vi "Main.vi"(10 "DAQ Type":enum16{"Hardware", "Simulation"}(ring), 11 "Module Admin":refnum<class "Delacor_lib_QMH_Module Admin.lvclass">) -> ()   [LabVIEW 2016, in "Environment Chamber.lvlib"]
doc: "This template is based off of the Queued Message Handler design pattern and the Queued Message Handler project template that ships with LabVIEW.\n\nThe main difference is that the queue is private to this module and communication between modules is performed via Broadcast and Request events.\n\nRequest events are wrapped in public API methods and are handled in the Event Handling Loop (EHL) of this VI. Any module can register for Broadcast events sent by this module. The EHL generates messages based on user interface actions.\n\nThe Message Handling Loop (MHL) processes messages generated by the EHL, or by other messages. The messages are string values, so new messages can be added easily to the Message Cases case structure in the MHL. Each message cluster can also provide an optional value for Message Data, which is a variant that can be converted to whatever message-specific data is required.\n_____\nBased on DQMH Project Template 6.1.0.94."
uses:
  Environment Chamber.lvlib
  <vilib>/Delacor/Delacor QMH/Libraries/Module Admin_class/Delacor_lib_QMH_Module Admin.lvclass
  Class/ARS-0220/ARS-0220.lvclass
  D:/common_ATE/Libraries/Environment Chamber/Class/Abstract/Abstract.lvclass
  Module Data--cluster.ctl
  Class/Abstract/Abstract.lvclass
  <vilib>/Delacor/Delacor QMH/Libraries/Message Queue_class/Delacor_lib_QMH_Message Queue.lvclass/Delacor_lib_QMH_Message Queue.ctl
  Stop Argument--cluster.ctl
  <vilib>/Delacor/Delacor QMH/Libraries/Module Admin_class/Delacor_lib_QMH_Module Admin.lvclass/Delacor_lib_QMH_Module Admin.ctl
  REQ Initialize Hardware Argument--cluster.ctl
  REQ Initialize Hardware (Reply Payload)--cluster.ctl
  REQ Configure Parameter Argument--cluster.ctl
  Configure Parameter.ctl
  REQ Acquire Data Argument--cluster.ctl
  REQ Acquire Humidity Argument--cluster.ctl
  REQ Close Ref Argument--cluster.ctl
  REQ Retry EC Argument--cluster.ctl
  <vilib>/Utility/miscctls.llb/LVPointTypeDef.ctl
  <vilib>/Delacor/Delacor QMH/Libraries/Message Queue_class/Delacor_lib_QMH_Enqueue Message (Single).vi
  <vilib>/Delacor/Delacor QMH/Libraries/Module Admin_class/Delacor_lib_QMH_Get External Launch.vi
  <vilib>/Utility/error.llb/Error Cluster From Error Code.vi
  <vilib>/ErrorRing/Error Ring.xnode
  <vilib>/Delacor/Delacor QMH/Libraries/Message Queue_class/Delacor_lib_QMH_Message Queue.lvclass
panel:
  in  "Acquire Humidity":bool
  out "error out":errorcluster
  out "Status":string
  in  "Simulate MHL Error":bool
  in  "Simulate EHL Error":bool
  # "Other QMH Modules communicate with this Module via its Public API (wrappers for its Request Events).\n\nThis Module communicates with other Modules via its Broadcast Events.\nAny module that wants to get these messages, just registers for this module's Broadcast events."
  # "This template is for the Delacor Modified Queued Message Handler design pattern.\n\nSee the block diagram for more information on how to use this template."
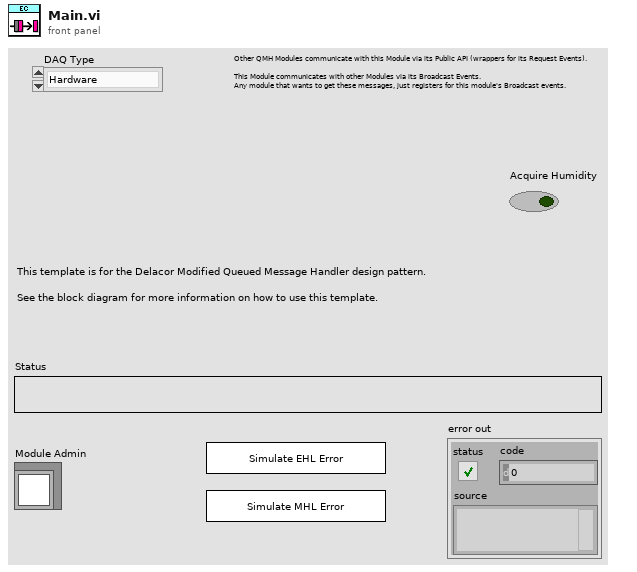
[diagram p1: front panel]
types:
  T1 = typedef "Environment Chamber.lvlib/Module Data--cluster.ctl" = cluster{"Status":string, "Abstract.lvclass":refnum<class "Abstract.lvclass">, "DAQ Type":enum16{"Hardware", "Simulation"}, "Connection Ref":variant}
  T2 = typedef "Environment Chamber.lvlib/Request Events--cluster.ctl" = cluster{"Stop Module":refnum<user-event>, "Show Panel":refnum<user-event>, "Hide Panel":refnum<user-event>, "Get Module Execution Status":refnum<user-event>, "Show Diagram":refnum<user-event>, "REQ Initialize Hardware":refnum<user-event>, "REQ Configure Parameter":refnum<user-event>, "REQ Acquire Data":refnum<user-event>, "REQ Acquire Humidity":refnum<user-event>, "REQ Close Ref":refnum<user-event>, "Broad Humidity Data":refnum<user-event>, "REQ Wakeup_helper_loop":refnum<user-event>, "REQ Retry EC":refnum<user-event>}
  T3 = enum32{"invalid lock state", "Not Locked", "Locked (No Password)", "Password-protected"}
  T4 = typedef "Environment Chamber.lvlib/Stop Argument--cluster.ctl" = cluster{"Origin":string, "Exit via Stop Module Req?":bool, "Wait for Module to stop?":bool}
  T5 = typedef "Environment Chamber.lvlib/REQ Initialize Hardware Argument--cluster.ctl" = cluster{"Connection Ref":variant, "Wait Notifier":refnum<notifier>, "wait for reply":bool}
  T6 = typedef "Environment Chamber.lvlib/REQ Configure Parameter Argument--cluster.ctl" = cluster{"Configure Parameter":T7}
  T7 = typedef "Environment Chamber.lvlib/Configure Parameter.ctl" = cluster{"Temp Parameter":cluster{"Temperature setpoint":dbl, "upper limit":dbl, "lower limit":dbl}, "Humidity Parameter":cluster{"Humidity setpoint":dbl, "upper limit":dbl, "lower limit":dbl}}
  T8 = typedef "Environment Chamber.lvlib/REQ Acquire Data Argument--cluster.ctl" = cluster{"Acquire Data":bool}
  T9 = typedef "Environment Chamber.lvlib/REQ Acquire Humidity Argument--cluster.ctl" = cluster{"Acquire Humidity":bool}
  T10 = typedef "Environment Chamber.lvlib/REQ Close Ref Argument--cluster.ctl" = cluster{"Boolean":bool}
  T11 = typedef "Environment Chamber.lvlib/REQ Retry EC Argument--cluster.ctl" = cluster{"Boolean":bool}
  T12 = typedef "LVPointTypeDef.ctl" = cluster{"Horizontal":i16, "Vertical":i16}
  T13 = enum32{"Invalid", "Standard", "Closed", "Hidden", "Minimized", "Maximized"}
  T14 = typedef "Environment Chamber.lvlib/REQ Initialize Hardware (Reply Payload)--cluster.ctl" = cluster{"Connect?":bool, "error":errorcluster}
  T15 = cluster{"measured humidity":dbl, "humidity setpoint":dbl, "upper limit alarm":dbl, "lower limit alarm":dbl}
  T16 = cluster{"measured temp":dbl, "temp setpoint":dbl, "upper limit alarm":dbl, "lower limit alarm":dbl}
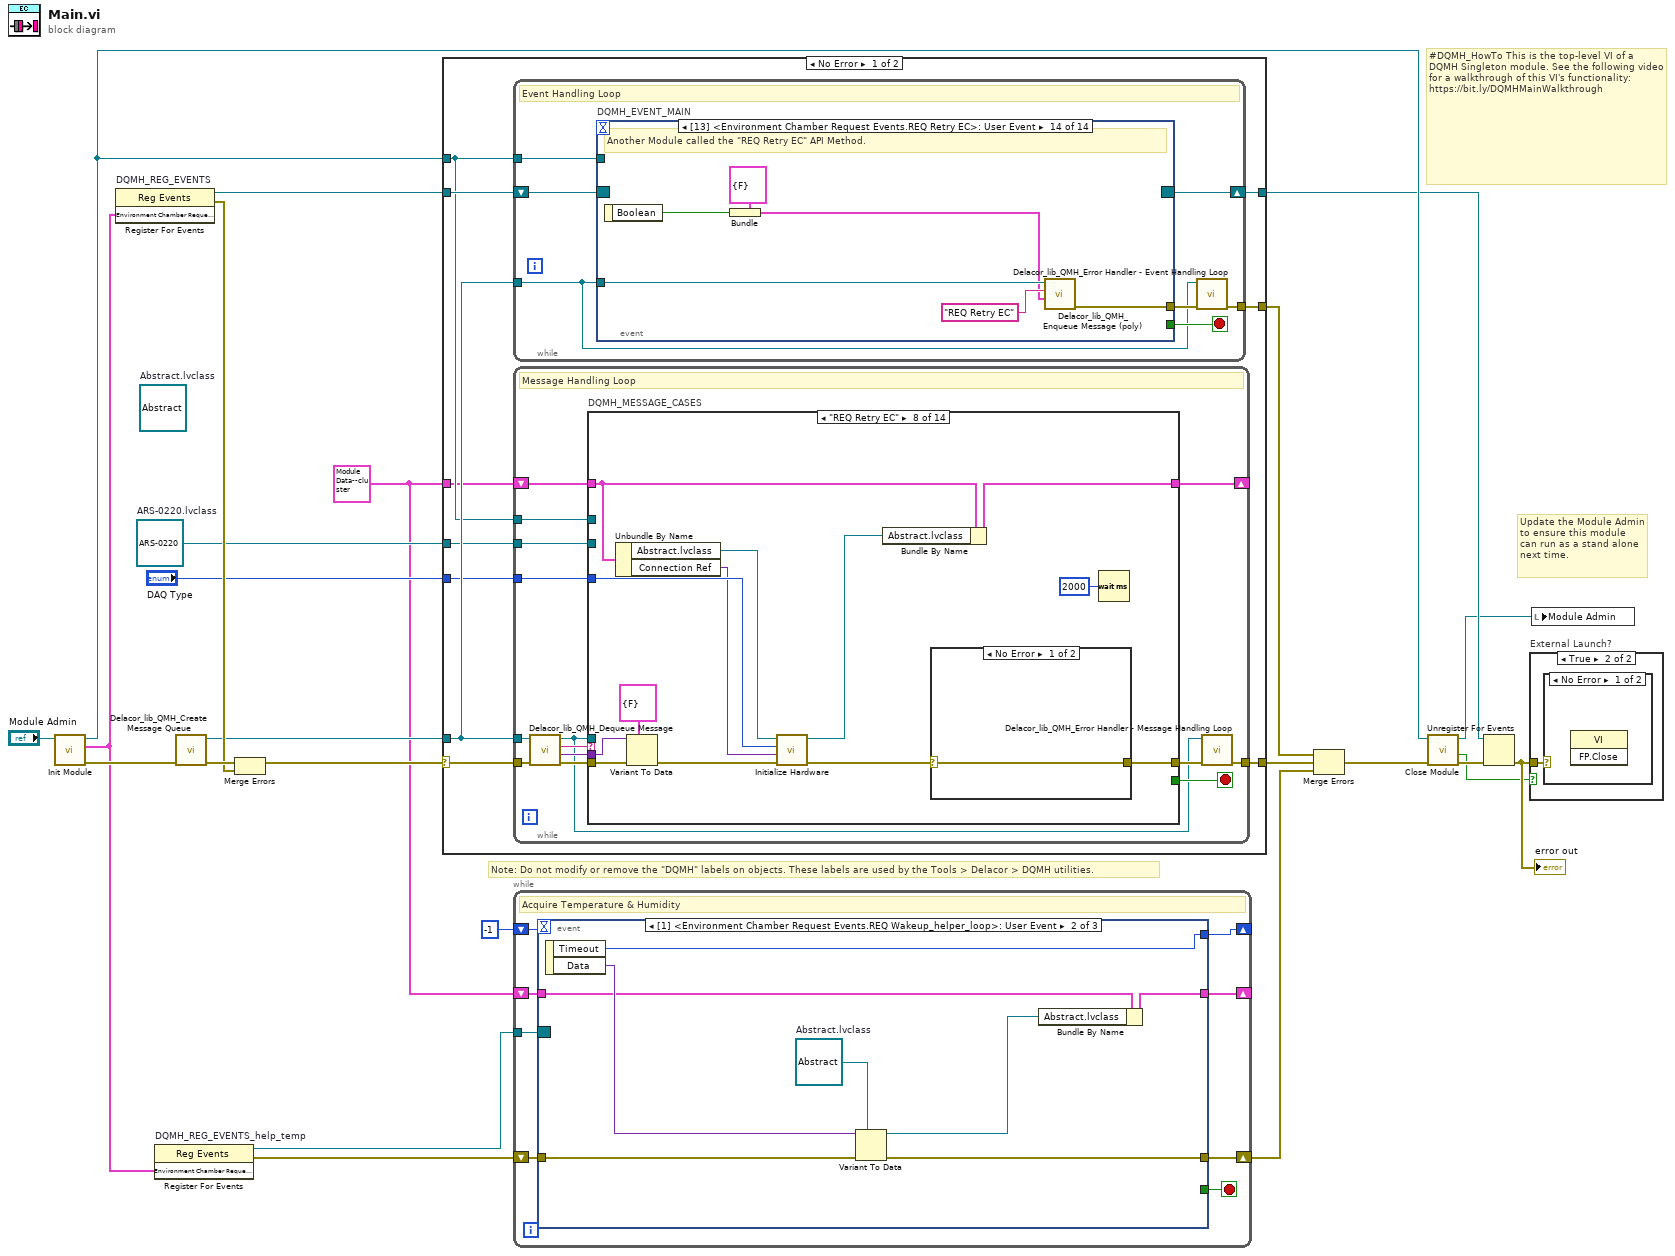
[diagram p0: block diagram]
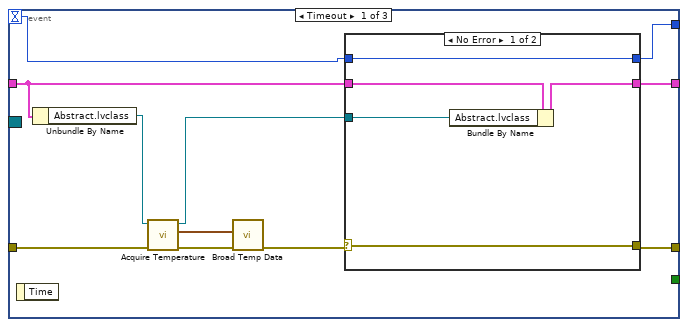
[diagram p2: hidden frame]
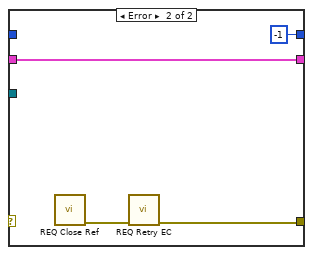
[diagram p3: hidden frame]
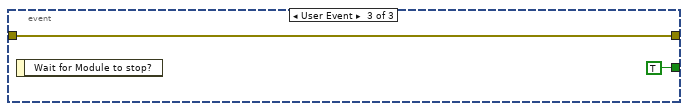
[diagram p4: hidden frame]
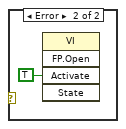
[diagram p6: hidden frame]
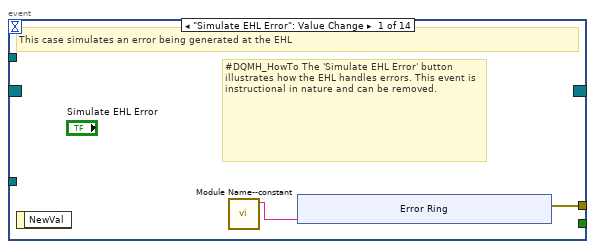
[diagram p7: hidden frame]
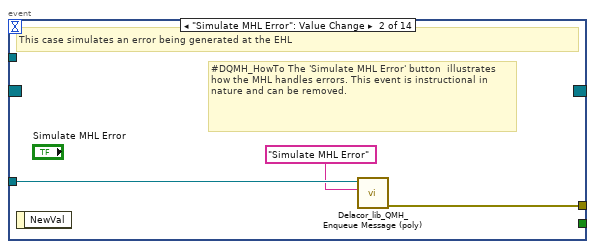
[diagram p8: hidden frame]
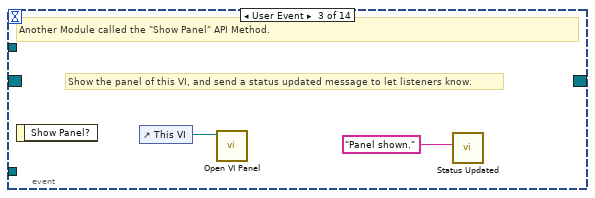
[diagram p9: hidden frame]
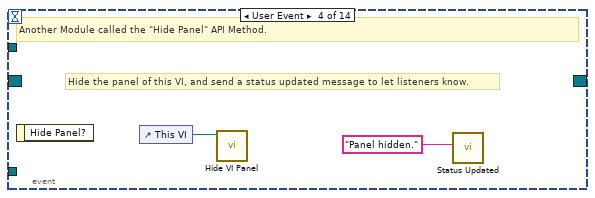
[diagram p10: hidden frame]
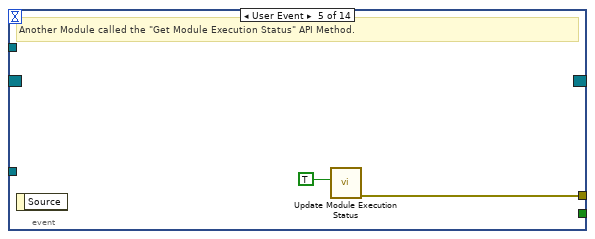
[diagram p11: hidden frame]
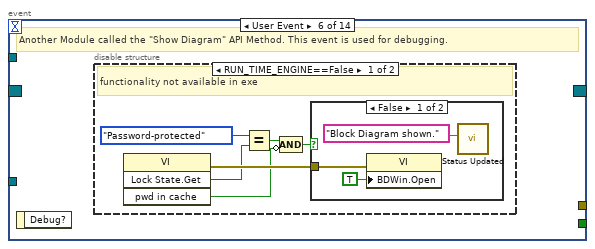
[diagram p12: hidden frame]
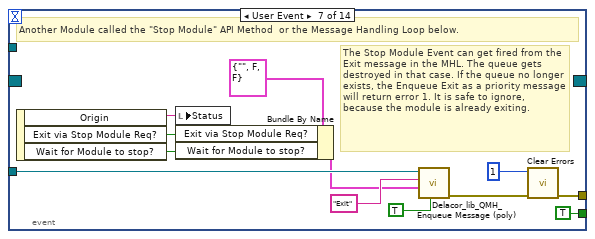
[diagram p15: hidden frame]
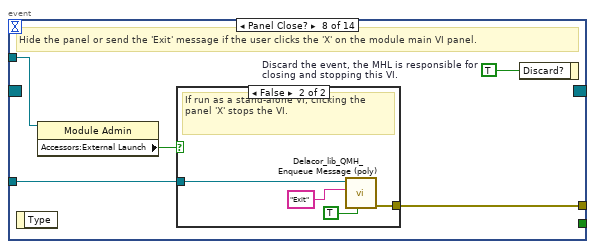
[diagram p16: hidden frame]
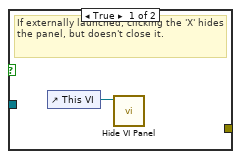
[diagram p17: hidden frame]
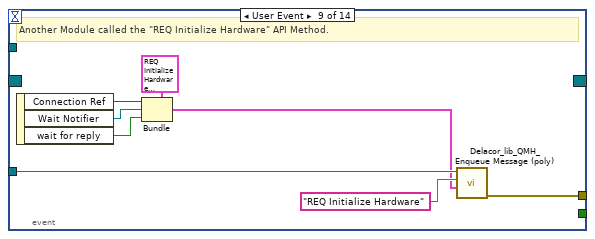
[diagram p18: hidden frame]
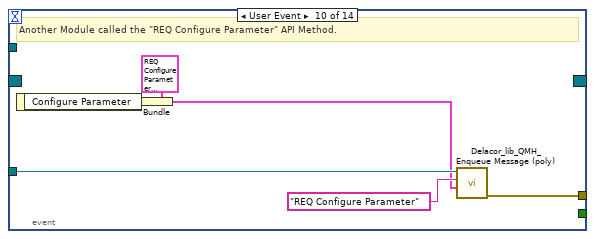
[diagram p19: hidden frame]
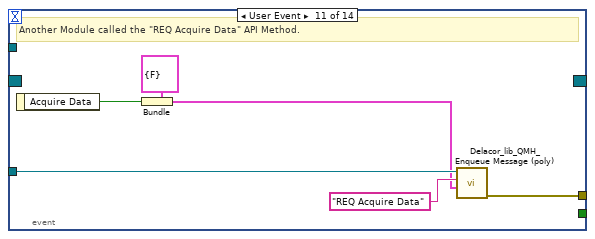
[diagram p20: hidden frame]
diagram:
  w1 = T1 {"Status"="", "Abstract.lvclass"=refnum, "DAQ Type"=enum."Hardware", "Connection Ref"=variant} ("Data Cluster")
  w8 = refnum<class "ARS-0220.lvclass"> refnum  # ARS-0220.lvclass
  (unwired) refnum<class "Abstract.lvclass"> refnum  # Abstract.lvclass
  # "#DQMH_HowTo This is the top-level VI of a DQMH Singleton module. See the following video for a walkthrough of this VI's functionality: https://bit.ly/DQMHMainWalkthrough"
  # "Note: Do not modify or remove the \"DQMH\" labels on objects. These labels are used by the Tools > Delacor > DQMH utilities."
  # "Update the Module Admin to ensure this module can run as a stand alone next time."
  n1 = call "Init Module.vi"("Singleton Module Admin in"="Module Admin") -> ("error out"=w23:errorcluster, "Environment Chamber Request Events"=w6:T2, "Singleton Module Admin out"=w15:refnum<class "Delacor_lib_QMH_Module Admin.lvclass">)  [unwired: 8 in]
  n2 = register-events "DQMH_REG_EVENTS"(w6) -> (reference out=w13:refnum<event-registration>, error out=w16:errorcluster)  [unwired: 2 in]
  n3 = register-events "DQMH_REG_EVENTS_help_temp"(w6) -> (reference out=w5:refnum<event-registration>, error out=w4:errorcluster)  [unwired: 2 in]
  n4 = call <vilib>:"Delacor_lib_QMH_Create Message Queue.vi"("error in"=w23) -> ("error out"=w18:errorcluster, "Message Queue"=w12:refnum<class "Delacor_lib_QMH_Message Queue.lvclass">)  [unwired: 9 in]
  n5 = Merge Errors(w18, w16) -> (w17:errorcluster)
  n6 = case shown="No Error" w17 {
    selector: w17 -> [w32 w317]
    tunnel: [w34 w316] -> w24
    tunnel: [w31 w322] -> w14
    tunnel: w13 -> [w30 w322]
    tunnel: w12 -> [w29 w315]
    tunnel: [w33 _] -> w21
    tunnel: w15 -> [w28 w318]
    tunnel: w8 -> [w27 _]
    tunnel: "DAQ Type" -> [w26 _]
    tunnel: w1 -> [w25 _]
    frame No Error {
      n7 = while {
        tunnel: w29 -> [w35]
        shift-right: [w38] -> w31
        shift-left: w30 -> [w39]
        tunnel: [w40] -> w33
        tunnel: w28 -> [w36]
        stop <- w37 stop-if-true
        # "Event Handling Loop"
        n8 = event "DQMH_EVENT_MAIN" shown="[13] <Environment Chamber Request Events.REQ Retry EC>: User Event" {
          selector: w39 -> [_ _ _ _ _ _ _ _ _ _ _ _ _ _]
          dyn-events: [_ _ _ _ _ _ _ _ _ _ _ _ _ _] -> w38
          timeout: _ -> [_ _ _ _ _ _ _ _ _ _ _ _ _ _]
          tunnel: [_ _ _ _ _ _ TRUE ("Discard?") _ _ _ _ _ _ _] -> w37
          tunnel: w35 -> [_ w52 _ _ _ _ w76 w83 w98 w104 w110 w116 w122 w128]
          tunnel: [w43 w53 _ _ w59 _ w79 w85 w91 w99 w105 w111 w117 w123] -> w41
          tunnel: w36 -> [_ _ _ _ _ _ _ w82 _ _ _ _ _ _]
          event "Simulate EHL Error": Value Change {
            # "#DQMH_HowTo The 'Simulate EHL Error' button  illustrates how the EHL handles errors. This event is instructional in nature and can be removed."
            # "This case simulates an error being generated at the EHL"
            n9 = event-data() -> ()  [unwired: 1 in, 1 out]
            n10 = call "Module Name--constant.vi"() -> ("Module Name"=w42:string)  [unwired: 11 in]
            n11 = xnode "Error Ring"("parameter 0"=w42) -> ("error out"=w43:errorcluster)
          }
          event "Simulate MHL Error": Value Change {
            # "#DQMH_HowTo The 'Simulate MHL Error' button  illustrates how the MHL handles errors. This event is instructional in nature and can be removed."
            # "This case simulates an error being generated at the EHL"
            n12 = event-data() -> ()  [unwired: 1 in, 1 out]
            n13 = call-poly <vilib>:"Delacor_lib_QMH_Enqueue Message (poly).vi"("Message"="Simulate MHL Error", "Message Queue in"=w52) -> ("error out"=w53:errorcluster)  [unwired: 8 in, 1 out]
          }
          event User Event {
            # "Show the panel of this VI, and send a status updated message to let listeners know."
            # "Another Module called the \"Show Panel\" API Method."
            n14 = event-data() -> ()  [unwired: 1 in, 1 out]
            n15 = control-ref of="This VI"() -> (w55:refnum<vi>)
            n16 = call "Open VI Panel.vi"("VI"=w55) -> ()  [unwired: 10 in, 1 out]
            n17 = call "Status Updated.vi"("Status"="Panel shown." ("format string")) -> ()  [unwired: 10 in, 1 out]
          }
          event User Event {
            # "Hide the panel of this VI, and send a status updated message to let listeners know."
            # "Another Module called the \"Hide Panel\" API Method."
            n18 = event-data() -> ()  [unwired: 1 in, 1 out]
            n19 = control-ref of="This VI"() -> (w57:refnum<vi>)
            n20 = call "Hide VI Panel.vi"("VI"=w57) -> ()  [unwired: 10 in, 1 out]
            n21 = call "Status Updated.vi"("Status"="Panel hidden." ("format string")) -> ()  [unwired: 10 in, 1 out]
          }
          event User Event {
            # "Another Module called the \"Get Module Execution Status\" API Method."
            n22 = event-data() -> ()  [unwired: 1 in, 1 out]
            n23 = call "Update Module Execution Status.vi"("Running?"=TRUE) -> ("error out"=w59:errorcluster)  [unwired: 10 in]
          }
          event User Event {
            # "Another Module called the \"Show Diagram\" API Method. This event is used for debugging."
            n24 = event-data() -> ()  [unwired: 1 in, 1 out]
            n25 = disable-structure shown="RUN_TIME_ENGINE==False" {
              frame condition #0 (active) {
                # "functionality not available in exe"
                n26 = invoke class="VI" method="Lock State.Get"() -> (error out=w65:errorcluster, "Get Lock State"=w64:T3, "pwd in cache"=w61:bool)  [unwired: 4 in, 1 out]
                n27 = Equal?(x=T3."Password-protected", y=w64) -> (x = y?=w62:bool)
                n28 = Compound Arithmetic op=AND(w62, invert w61) -> (w60:bool)
                n29 = case shown="False" w60 {
                  tunnel: w65 -> [w68 _]
                  frame False {
                    n30 = property class="VI"(error in=w68, "BDWin.Open"=TRUE ("Block Diagram Window:Open")) -> ()  [unwired: 1 in, 2 out]
                    n31 = call "Status Updated.vi"("Status"="Block Diagram shown." ("format string")) -> ()  [unwired: 10 in, 1 out]
                  }
                  frame True {
                    # "Password-protected VI, and the password is not in the cache. Do not show the diagram."
                  }
                }
              }
              frame condition #1 {
              }
            }
          }
          event User Event {
            # "The Stop Module Event can get fired from the Exit message in the MHL. The queue gets destroyed in that case. If the queue no longer exists, the Enqueue Exit as a priority message will return error 1. It is safe to ignore, because the module is already exiting."
            # "Another Module called the \"Stop Module\" API Method  or the Message Handling Loop below."
            n32 = event-data() -> ("Origin"=w75:string, "Exit via Stop Module Req?"=w71:bool, "Wait for Module to stop?"=w70:bool)  [unwired: 1 in]
            n33 = local write "Status"(w75) -> ()
            n34 = Bundle By Name(cluster=T4 {"Origin"="", "Exit via Stop Module Req?"=FALSE, "Wait for Module to stop?"=FALSE} ("Stop Argument"), "Exit via Stop Module Req?"=w71, "Wait for Module to stop?"=w70) -> (w69:T4)
            n35 = call-poly <vilib>:"Delacor_lib_QMH_Enqueue Message (poly).vi"("Priority Message? (F)"=TRUE, "Message Data"=w69, "Message"="Exit", "Message Queue in"=w76) -> ("error out"=w80:errorcluster)  [unwired: 6 in, 1 out]
            n36 = call <vilib>:"Clear Errors.vi"("error in (no error)"=w80, "specific error code to clear (0: all)"=1) -> ("error out"=w79:errorcluster)  [unwired: 4 in, 1 out]
          }
          event Panel Close? {
            w84 = TRUE  # Discard the event, the MHL is responsible for closing and stopping this VI.
            # "Hide the panel or send the 'Exit' message if the user clicks the 'X' on the module main VI panel."
            n37 = event-data() -> ()  [unwired: 1 in, 1 out]
            n38 = property class="Module Admin"(reference=w82) -> ("Accessors:External Launch"=w81:bool)  [unwired: 1 in, 2 out]
            n39 = case shown="False" w81 {
              tunnel: w83 -> [_ w89]
              tunnel: [_ w90] -> w85
              frame True {
                # "If externally launched, clicking the 'X' hides the panel, but doesn't close it."
                n40 = control-ref of="This VI"() -> (w86:refnum<vi>)
                n41 = call "Hide VI Panel.vi"("VI"=w86) -> ()  [unwired: 10 in, 1 out]
              }
              frame False {
                # "If run as a stand-alone VI, clicking the panel 'X' stops the VI."
                n42 = call-poly <vilib>:"Delacor_lib_QMH_Enqueue Message (poly).vi"("Priority Message? (F)"=TRUE, "Message"="Exit", "Message Queue in"=w89) -> ("error out"=w90:errorcluster)  [unwired: 7 in, 1 out]
              }
            }
            n43 = event-data("Discard?"=w84) -> ()  [unwired: 1 in, 1 out]
          }
          event User Event {
            # "Another Module called the \"REQ Initialize Hardware\" API Method."
            n44 = event-data() -> ("Connection Ref"=w94:variant, "Wait Notifier"=w93:refnum<notifier>, "wait for reply"=w92:bool)  [unwired: 1 in]
            n45 = Bundle(cluster=T5 {"Connection Ref"=variant, "Wait Notifier"=refnum, "wait for reply"=FALSE} ("REQ Initialize Hardware Argument"), "Connection Ref"=w94, "Wait Notifier"=w93, "wait for reply"=w92) -> (w95:T5)
            n46 = call-poly <vilib>:"Delacor_lib_QMH_Enqueue Message (poly).vi"("Message Data"=w95, "Message"="REQ Initialize Hardware", "Message Queue in"=w98) -> ("error out"=w91:errorcluster)  [unwired: 7 in, 1 out]
          }
          event User Event {
            # "Another Module called the \"REQ Configure Parameter\" API Method."
            n47 = event-data() -> ("Configure Parameter"=w100:T7)  [unwired: 1 in]
            n48 = Bundle(cluster=T6 {"Configure Parameter"={"Temp Parameter"={"Temperature setpoint"=40.0, "upper limit"=80.0, "lower limit"=0.0}, "Humidity Parameter"={"Humidity setpoint"=50.0, "upper limit"=80.0, "lower limit"=0.0}}} ("REQ Configure Parameter Argument"), "Configure Parameter"=w100) -> (w101:T6)
            n49 = call-poly <vilib>:"Delacor_lib_QMH_Enqueue Message (poly).vi"("Message Data"=w101, "Message"="REQ Configure Parameter", "Message Queue in"=w104) -> ("error out"=w99:errorcluster)  [unwired: 7 in, 1 out]
          }
          event User Event {
            # "Another Module called the \"REQ Acquire Data\" API Method."
            n50 = event-data() -> ("Acquire Data"=w106:bool)  [unwired: 1 in]
            n51 = Bundle(cluster=T8 {"Acquire Data"=FALSE} ("REQ Acquire Data Argument"), "Acquire Data"=w106) -> (w107:T8)
            n52 = call-poly <vilib>:"Delacor_lib_QMH_Enqueue Message (poly).vi"("Message Data"=w107, "Message"="REQ Acquire Data", "Message Queue in"=w110) -> ("error out"=w105:errorcluster)  [unwired: 7 in, 1 out]
          }
          event User Event {
            # "Another Module called the \"REQ Acquire Humidity\" API Method."
            n53 = event-data() -> ("Acquire Humidity"=w112:bool)  [unwired: 1 in]
            n54 = Bundle(cluster=T9 {"Acquire Humidity"=FALSE} ("REQ Acquire Humidity Argument"), "Acquire Humidity"=w112) -> (w113:T9)
            n55 = call-poly <vilib>:"Delacor_lib_QMH_Enqueue Message (poly).vi"("Message Data"=w113, "Message"="REQ Acquire Humidity", "Message Queue in"=w116) -> ("error out"=w111:errorcluster)  [unwired: 7 in, 1 out]
          }
          event User Event {
            # "Another Module called the \"REQ Close Ref\" API Method."
            n56 = event-data() -> ("Boolean"=w118:bool)  [unwired: 1 in]
            n57 = Bundle(cluster=T10 {"Boolean"=FALSE} ("REQ Close Ref Argument"), "Boolean"=w118) -> (w119:T10)
            n58 = call-poly <vilib>:"Delacor_lib_QMH_Enqueue Message (poly).vi"("Message Data"=w119, "Message"="REQ Close Ref", "Message Queue in"=w122) -> ("error out"=w117:errorcluster)  [unwired: 7 in, 1 out]
          }
          event User Event {
            # "Another Module called the \"REQ Retry EC\" API Method."
            n59 = event-data() -> ("Boolean"=w124:bool)  [unwired: 1 in]
            n60 = Bundle(cluster=T11 {"Boolean"=FALSE} ("REQ Retry EC Argument"), "Boolean"=w124) -> (w125:T11)
            n61 = call-poly <vilib>:"Delacor_lib_QMH_Enqueue Message (poly).vi"("Message Data"=w125, "Message"="REQ Retry EC", "Message Queue in"=w128) -> ("error out"=w123:errorcluster)  [unwired: 7 in, 1 out]
          }
        }
        n62 = call-dynamic "Delacor_lib_QMH_Error Handler - Event Handling Loop.vi"("error in"=w41, "Message Queue in"=w35) -> ("dup error in"=w40:errorcluster)  [unwired: 8 in, 1 out]
      }
      n63 = while {
        tunnel: w29 -> [w133]
        shift-right: [w137] -> _
        shift-left: w25 -> [w138]
        tunnel: w32 -> [w141]
        tunnel: [w139] -> w34
        tunnel: w28 -> [w131]
        tunnel: w27 -> [w130]
        tunnel: w26 -> [w129]
        stop <- w136 stop-if-true
        # "Message Handling Loop"
        n64 = call-dynamic "Delacor_lib_QMH_Dequeue Message.vi"("error in"=w141, "Message Queue in"=w133) -> ("error out"=w140:errorcluster, "Message Data"=w134:variant, "Message"=w135:string, "Message Queue out"=w132:refnum<class "Delacor_lib_QMH_Message Queue.lvclass">)  [unwired: 6 in]
        n65 = case "DQMH_MESSAGE_CASES" shown="\"REQ Retry EC\"" w135 {
          selector: w135 -> [_ _ _ _ _ _ _ _ _ _ _ _ _ w302]
          tunnel: w132 -> [_ _ _ _ _ _ _ _ _ _ _ w272 w295 _]
          tunnel: w140 -> [w162 w166 w184 w197 w210 w224 w237 w250 w255 w257 w262 w279 w286 w304]
          tunnel: [w160 w166 w171 w192 w200 w215 w233 w239 w254 w257 w261 w275 w298 w305] -> w142
          tunnel: w138 -> [w151 w165 w175 w191 w205 w220 w232 w246 w253 w256 w259 w274 w294 w303]
          tunnel: [w150 w165 w172 w189 w203 w218 w230 w242 w253 w256 w259 w274 w294 w303] -> w137
          tunnel: [_ _ _ _ _ _ _ _ _ _ _ _ w293 _] -> w136
          tunnel: w134 -> [_ _ w183 w196 w209 w223 w236 w249 _ _ _ w273 w292 _]
          tunnel: w131 -> [w152 _ _ _ _ _ _ _ _ _ _ w271 w287 _]
          tunnel: w130 -> [w145 _ _ _ _ _ _ _ _ _ _ _ _ _]
          tunnel: w129 -> [w143 _ _ _ _ _ _ w244 _ _ _ _ _ _]
          frame "Initialize" {
            w144 = "Initial Message" ("Initial Message")
            # "Initialize - Any operation that needs to be done before the module can receive messages. Synchronize Caller Events.vi will inform Start Module.vi that the module has launched and is ready to receive messages. Module Did Init.vi will broadcast that the module initialized."
            n66 = call "Synchronize Caller Events.vi"("error in (no error)"=w162, "Singleton Module Admin in"=w152) -> ("error out"=w161:errorcluster, "Singleton Module Admin out"=w147:refnum<class "Delacor_lib_QMH_Module Admin.lvclass">)  [unwired: 8 in]
            n67 = property class="Module Admin"(reference=w147) -> ("Accessors:External Launch"=w156:bool)  [unwired: 1 in, 2 out]
            n68 = Select(t=T13."Hidden" ("State"), s=w156, f=T13."Standard" ("State")) -> (s? t:f=w153:T13)
            n69 = call "Module Name--constant.vi"() -> ("Module Name"=w159:string)  [unwired: 11 in]
            n70 = property class="VI"("Front Panel.Title"=w159) -> (reference out=w158:refnum<vi>, error out=w164:errorcluster)  [unwired: 2 in]
            n71 = call "Module Name--constant.vi"() -> ("Module Name"=w148:string)  [unwired: 11 in]
            n72 = Bundle By Name(cluster=w151, "Status"=w144, "Abstract.lvclass"=w145, "DAQ Type"=w143) -> (w150:T1)
            n73 = invoke class="VI" method="FP.Open"(reference=w158, error in=w164, "State"=w153) -> (reference out=w157:refnum<vi>, error out=w163:errorcluster)  [unwired: 2 in, 3 out]
            n74 = call "Module Did Init.vi"("error in (no error)"=w161, "Initialized?"=TRUE, "Origin"=w148) -> ("error out"=w160:errorcluster)  [unwired: 8 in]
            n75 = invoke class="VI" method="FP.Center"(reference=w157, error in=w163) -> ()  [unwired: 1 in, 3 out]
            n76 = property on="Pane" class="Pane"("Origin"=T12 {"Horizontal"=0, "Vertical"=0}) -> ()  [unwired: 2 in, 2 out]
            "Status" <- w144
          }
          frame "---Module Specific---" {
            # "Separator -- The following cases handle messages specific to this Module."
          }
          frame "REQ Initialize Hardware" {
            n77 = Variant To Data(error in=w184, type=T5 {"Connection Ref"=variant, "Wait Notifier"=refnum, "wait for reply"=FALSE} ("REQ Initialize Hardware Argument"), Variant=w183) -> (data=w181:T5, error out=w176:errorcluster)
            n78 = Unbundle By Name(w175) -> ("Abstract.lvclass"=w174:refnum<class "Abstract.lvclass">, "DAQ Type"=w173:enum16{"Hardware", "Simulation"})
            n79 = Unbundle By Name(w181) -> ("Wait Notifier"=w180:refnum<notifier>, "wait for reply"=w179:bool, "Connection Ref"=w167:variant)
            n80 = call-dynamic "Initialize Hardware.vi"("error in (no error)"=w176, "Connection Ref"=w167, "DAQ Type"=w173, "Abstract in"=w174) -> ("error out"=w171:errorcluster, "Abstract out"=w168:refnum<class "Abstract.lvclass">)  [unwired: 6 in]
            n81 = Unbundle By Name(w171) -> ("status"=w170:bool)
            n82 = Not(x=w170) -> (.not. x?=w169:bool)
            n83 = Bundle By Name(cluster=w175, "Connection Ref"=w167, "Abstract.lvclass"=w168) -> (w172:T1)
            n84 = Bundle By Name(cluster=T14 {"Connect?"=FALSE, "error"={"status"=FALSE, "code"=0, "source"=""}} ("REQ Initialize Hardware (Reply Payload)"), "Connect?"=w169) -> (w178:T14)
            n85 = case shown="True" w179 {
              tunnel: w180 -> [_ w186]
              tunnel: w178 -> [_ w185]
              frame False {
              }
              frame True {
                n86 = Send Notification(notification=w185, notifier=w186) -> ()  [unwired: 1 in, 2 out]
              }
            }
          }
          frame "REQ Configure Parameter" {
            n87 = Variant To Data(error in=w197, type=T6 {"Configure Parameter"={"Temp Parameter"={"Temperature setpoint"=40.0, "upper limit"=80.0, "lower limit"=0.0}, "Humidity Parameter"={"Humidity setpoint"=50.0, "upper limit"=80.0, "lower limit"=0.0}}} ("REQ Configure Parameter Argument"), Variant=w196) -> (data=w194:T6, error out=w193:errorcluster)
            n88 = Unbundle By Name(w194) -> ("Configure Parameter"=w187:T7)
            n89 = Unbundle By Name(w191) -> ("Abstract.lvclass"=w190:refnum<class "Abstract.lvclass">)
            n90 = call-dynamic "Configure Parameter.vi"("error in (no error)"=w193, "Configure Parameter"=w187, "Abstract in"=w190) -> ("error out"=w192:errorcluster, "Abstract out"=w188:refnum<class "Abstract.lvclass">)  [unwired: 7 in]
            n91 = Bundle By Name(cluster=w191, "Abstract.lvclass"=w188) -> (w189:T1)
          }
          frame "REQ Acquire Data" {
            n92 = Variant To Data(error in=w210, type=T8 {"Acquire Data"=FALSE} ("REQ Acquire Data Argument"), Variant=w209) -> (data=w207:T8, error out=w206:errorcluster)
            n93 = Unbundle By Name(w205) -> ("Abstract.lvclass"=w204:refnum<class "Abstract.lvclass">)
            n94 = Unbundle By Name(w207) -> ("Acquire Data"=w202:bool)
            n95 = call-dynamic "Acquire Data.vi"("error in (no error)"=w206, "Acquire Data"=w202, "Abstract in"=w204) -> ("error out"=w201:errorcluster, "Abstract out"=w199:refnum<class "Abstract.lvclass">)  [unwired: 7 in]
            n96 = Bundle By Name(cluster=w205, "Abstract.lvclass"=w199) -> (w203:T1)
            n97 = call "REQ Wakeup_helper_loop.vi"("error in"=w201, "Timeout"=0, "Data"=w199) -> ("error out"=w200:errorcluster)  [unwired: 8 in]
          }
          frame "REQ Acquire Humidity" {
            n98 = Variant To Data(error in=w224, type=T9 {"Acquire Humidity"=FALSE} ("REQ Acquire Humidity Argument"), Variant=w223) -> (data=w221:T9, error out=w216:errorcluster)
            n99 = Unbundle By Name(w221) -> ("Acquire Humidity"=w214:bool)
            n100 = Unbundle By Name(w220) -> ("Abstract.lvclass"=w219:refnum<class "Abstract.lvclass">)
            n101 = call-dynamic "Acquire Humidity.vi"("error in (no error)"=w216, "Abstract in"=w219) -> ("error out"=w213:errorcluster, "Humidity Data"=w211:T15, "Abstract out"=w217:refnum<class "Abstract.lvclass">)  [unwired: 7 in]
            n102 = Bundle By Name(cluster=w220, "Abstract.lvclass"=w217) -> (w218:T1)
            n103 = call "Broad Humidity. Data.vi"("error in"=w213, "Humidity Data"=w211) -> ("error out"=w212:errorcluster)  [unwired: 9 in]
            n104 = case shown="No Error" w212 {
              selector: w212 -> [w227 w228]
              tunnel: [w226 w228] -> w215
              tunnel: w214 -> [w225 _]
              frame No Error {
                n105 = property on="Acquire Humidity" class="Bool (strict)"(error in=w227, "Val(Sgnl)"=w225) -> (error out=w226:errorcluster)  [unwired: 1 in, 1 out]
              }
              frame Error {
              }
            }
          }
          frame "REQ Close Ref" {
            (unwired) FALSE ("Value (Signaling)")
            n106 = Variant To Data(error in=w237, type=T10 {"Boolean"=FALSE} ("REQ Close Ref Argument"), Variant=w236) -> (data=w234:T10)  [unwired: 1 out]
            n107 = Unbundle By Name(w234) -> ()  [unwired: 1 out]
            n108 = Unbundle By Name(w232) -> ("Abstract.lvclass"=w231:refnum<class "Abstract.lvclass">)
            n109 = call-dynamic "Close Ref.vi"("Abstract in"=w231) -> ("error out"=w233:errorcluster, "Abstract out"=w229:refnum<class "Abstract.lvclass">)  [unwired: 9 in]
            n110 = Bundle By Name(cluster=w232, "Abstract.lvclass"=w229) -> (w230:T1)
          }
          frame "REQ Retry EC" {
            n111 = Unbundle By Name(w246) -> ("Abstract.lvclass"=w245:refnum<class "Abstract.lvclass">, "Connection Ref"=w243:variant)
            n112 = Variant To Data(error in=w250, type=T11 {"Boolean"=FALSE} ("REQ Retry EC Argument"), Variant=w249) -> (error out=w247:errorcluster)  [unwired: 1 out]
            n113 = call-dynamic "Initialize Hardware.vi"("error in (no error)"=w247, "Connection Ref"=w243, "DAQ Type"=w244, "Abstract in"=w245) -> ("error out"=w240:errorcluster, "Abstract out"=w241:refnum<class "Abstract.lvclass">)  [unwired: 6 in]
            n114 = Bundle By Name(cluster=w246, "Abstract.lvclass"=w241) -> (w242:T1)
            n115 = case shown="No Error" w240 {
              selector: w240 -> [w251 _]
              tunnel: [w251 w252] -> w239
              frame No Error {
              }
              frame Error {
                n116 = call "REQ Retry EC.vi"() -> ("error out"=w252:errorcluster)  [unwired: 11 in]
              }
            }
            n117 = Wait (ms)(milliseconds to wait=u32 2000) -> ()  [unwired: 1 out]
          }
          frame "---Copy This Frame---" {
            # "Duplicate this frame when creating new messages.  Change this comment in the duplicated frame to describe this message."
            n118 = Merge Errors(w255) -> (w254:errorcluster)
          }
          frame "---Exit and Error Handling---" {
            # "Separator - The following cases handle errors and exit messages."
          }
          frame "Simulate MHL Error" {
            # "#DQMH_HowTo The 'Simulate MHL Error' button  illustrates how the MHL handles errors. This event is instructional in nature and can be removed."
            # "Simulate an error occurring at the MHL"
            n119 = call "Module Name--constant.vi"() -> ("Module Name"=w258:string)  [unwired: 11 in]
            n120 = xnode "Error Ring"("parameter 0"=w258) -> ("error out"=w260:errorcluster)
            n121 = Merge Errors(w262, w260) -> (w261:errorcluster)
          }
          frame "Error" {
            # "#CodeRecommended - If you ever change the name of this \"Error\" message, you'll need to update the name in the Check Loop Error.vi as well."
            # "#CodeRecommended - If the module is running in standalone mode (External Launch = FALSE), this code will pop up an error dialog and call the 'Exit' message if an error occurs. Add more fine-grained error handling here."
            # "Error - Check the error message data and respond accordingly. This message is sent by the \"Error Handler\" VIs at the end of each loop in this application."
            n122 = property class="Module Admin"(reference=w271) -> ("Accessors:External Launch"=w270:bool)  [unwired: 1 in, 2 out]
            n123 = Variant To Data(error in=w279, type=errorcluster {"status"=FALSE, "code"=0, "source"=""} ("error constant"), Variant=w273) -> (data=w280:errorcluster, error out=w277:errorcluster)
            n124 = call "Error Reported.vi"("Error"=w280) -> ()  [unwired: 10 in, 1 out]
            n125 = case shown="False" w270 {
              tunnel: [w285 _] -> w276
              tunnel: w272 -> [w283 _]
              tunnel: w280 -> [w284 _]
              frame False {
                # "If the module is running standalone, then pop up an error dialog and call the \"Exit\" message."
                n126 = call <vilib>:"Simple Error Handler.vi"("error in (no error)"=w284) -> ()  [unwired: 4 in, 5 out]
                n127 = call-poly <vilib>:"Delacor_lib_QMH_Enqueue Message (poly).vi"("Priority Message? (F)"=TRUE, "Message"="Exit", "Message Queue in"=w283) -> ("error out"=w285:errorcluster)  [unwired: 7 in, 1 out]
              }
              frame True {
                # "If the module was launched externally, calling the Error Reported broadcast VI is the only action performed by the \"Error\" message. The module's caller can then process the error appropriately."
              }
            }
            n128 = Merge Errors(w277, w276) -> (w275:errorcluster)
            n129 = local write "error out"(w275) -> ()
          }
          frame "Exit" {
            w291 = 91  # 91: not all Exit messages will have an argument
            w293 = TRUE  # Stop the VI
            # "Release the message queue reference"
            # "#CodeNeeded - Add any required cleanup code here"
            # "Exit - Exit the application."
            n130 = Variant To Data(error in=w286, type=T4 {"Origin"="", "Exit via Stop Module Req?"=FALSE, "Wait for Module to stop?"=FALSE} ("Stop Argument"), Variant=w292) -> (data=w289:T4, error out=w297:errorcluster)
            n131 = call <vilib>:"Clear Errors.vi"("error in (no error)"=w297, "specific error code to clear (0: all)"=w291) -> ("error out"=w300:errorcluster)  [unwired: 4 in, 1 out]
            n132 = control-ref of="This VI"() -> (w288:refnum<vi>)
            n133 = call-dynamic "Delacor_lib_QMH_Release Message Queue.vi"("error in"=w300, "Message Queue"=w295) -> ("error out"=w299:errorcluster)  [unwired: 9 in]
            n134 = call "Handle Exit.vi"("Stop Argument"=w289, "Admin in"=w287, "VI reference"=w288) -> ("error out"=w296:errorcluster)  [unwired: 7 in, 1 out]
            n135 = Merge Errors(w299, w296) -> (w298:errorcluster)
          }
          frame Default {
            # "'Default' case only runs if there is a message that isn't defined in any of the other cases.  Output a programming error."
            n136 = call "Module Name--constant.vi"() -> ("Module Name"=w301:string)  [unwired: 11 in]
            n137 = xnode "Error Ring"("parameter 0"=w302, "parameter 1"=w301) -> ("error out"=w306:errorcluster)
            n138 = Merge Errors(w304, w306) -> (w305:errorcluster)
          }
        }
        n139 = call-dynamic "Delacor_lib_QMH_Error Handler - Message Handling Loop.vi"("error in"=w142, "Message Queue in"=w132) -> ("dup error in"=w139:errorcluster)  [unwired: 8 in, 1 out]
      }
    }
    frame Error {
      # "Synchronize Caller Events.vi will inform Start Module.vi that the module has launched and will let the code calling Start Module.vi register for broadcasts and would permit the caller receive the broadcast that an error occurred at launch time."
      n140 = call-dynamic "Delacor_lib_QMH_Release Message Queue.vi"("error in"=w317, "Message Queue"=w315) -> ("error out"=w316:errorcluster)  [unwired: 9 in]
      n141 = call "Synchronize Caller Events.vi"("Singleton Module Admin in"=w318) -> ("error out"=w323:errorcluster)  [unwired: 9 in, 1 out]
      n142 = call "Module Name--constant.vi"() -> ("Module Name"=w321:string)  [unwired: 11 in]
      n143 = Format Into String(format string="An error occurred during initialization. %s is no longer running.", w321) -> (resulting string=w319:string)  [unwired: 2 in, 1 out]
      n144 = Merge Errors(w316, w323) -> (w324:errorcluster)
      n145 = call "Error Reported.vi"("Additional Information"=w319, "Error"=w324) -> ()  [unwired: 9 in, 1 out]
    }
  }
  n146 = while {
    tunnel: w5 -> [w332]
    shift-right: [w327] -> _
    shift-left: -1 -> [w328]
    shift-right: [w329] -> w3
    shift-left: w4 -> [w331]
    shift-right: [w325] -> _
    shift-left: w1 -> [w326]
    stop <- w330 stop-if-true
    # "Acquire Temperature & Humidity"
    n147 = event shown="[1] <Environment Chamber Request Events.REQ Wakeup_helper_loop>: User Event" {
      selector: w332 -> [_ _ _]
      dyn-events: _ -> [_ _ _]
      timeout: w328 -> [w338 _ _]
      tunnel: w331 -> [w343 w359 w362]
      tunnel: [_ _ TRUE ("Wait for Module to stop?")] -> w330
      tunnel: [w333 w353 w362] -> w329
      tunnel: [w337 w360 _] -> w327
      tunnel: w326 -> [w336 w356 _]
      tunnel: [w335 w355 _] -> w325
      event Timeout {
        n148 = event-data() -> ()  [unwired: 1 in, 1 out]
        n149 = Unbundle By Name(w336) -> ("Abstract.lvclass"=w340:refnum<class "Abstract.lvclass">)
        n150 = call-dynamic "Acquire Temperature.vi"("error in (no error)"=w343, "Abstract in"=w340) -> ("error out"=w342:errorcluster, "Temp Data"=w341:T16, "Abstract out"=w334:refnum<class "Abstract.lvclass">)  [unwired: 7 in]
        n151 = call "Broad Temp Data.vi"("error in"=w342, "Temp Data"=w341) -> ("error out"=w339:errorcluster)  [unwired: 9 in]
        n152 = case shown="No Error" w339 {
          selector: w339 -> [w344 _]
          tunnel: w338 -> [w348 _]
          tunnel: [w348 -1] -> w337
          tunnel: w336 -> [w347 w351]
          tunnel: [w346 w351] -> w335
          tunnel: w334 -> [w345 _]
          tunnel: [w344 w349] -> w333
          frame No Error {
            n153 = Bundle By Name(cluster=w347, "Abstract.lvclass"=w345) -> (w346:T1)
          }
          frame Error {
            n154 = call "REQ Close Ref.vi"() -> ("error out"=w350:errorcluster)  [unwired: 11 in]
            n155 = call "REQ Retry EC.vi"("error in"=w350) -> ("error out"=w349:errorcluster)  [unwired: 10 in]
          }
        }
      }
      event User Event {
        w358 = refnum<class "Abstract.lvclass"> refnum  # Abstract.lvclass
        n156 = event-data() -> ("Timeout"=w360:i32, "Data"=w357:variant)  [unwired: 1 in]
        n157 = Variant To Data(error in=w359, type=w358, Variant=w357) -> (data=w354:refnum<class "Abstract.lvclass">, error out=w353:errorcluster)
        n158 = Bundle By Name(cluster=w356, "Abstract.lvclass"=w354) -> (w355:T1)
      }
      event User Event {
        n159 = event-data() -> ()  [unwired: 1 in, 1 out]
      }
    }
  }
  n160 = Merge Errors(w21, w24, w3) -> (w20:errorcluster)
  n161 = call "Close Module.vi"("error in (no error)"=w20, "Module Admin in"=w15) -> ("error out"=w22:errorcluster, "External Launch"=w9:bool, "Module Admin out"=w10:refnum<class "Delacor_lib_QMH_Module Admin.lvclass">)  [unwired: 7 in]
  n162 = Unregister For Events(event registration refnum=w14, error in=w22) -> (error out=w19:errorcluster)
  "error out" <- w19
  n163 = case "External Launch?" shown="True" w9 {
    tunnel: w19 -> [_ w363]
    frame False {
    }
    frame True {
      n164 = case shown="No Error" w363 {
        frame No Error {
          n165 = invoke class="VI" method="FP.Close"() -> ()  [unwired: 3 in, 3 out]
        }
        frame Error {
          n166 = invoke class="VI" method="FP.Open"("Activate"=TRUE ("Activate?")) -> ()  [unwired: 4 in, 5 out]
        }
      }
    }
  }
  n167 = local write "Module Admin"(w10) -> ()
